vi "CIClose.vi"(11 "Camera data":variant) -> ()   [LabVIEW 2011]
uses:
  mkCameraData.ctl
  CameraConfig.ctl
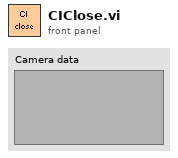
[diagram p1: front panel]
types:
  T1 = typedef "mkCameraData.ctl" = cluster{"Session":refnum<k11>, "Settings":T2}
  T2 = typedef "CameraConfig.ctl" = cluster{"Gain [1-4]":sgl, "Offset":i16, "Mode":i16, "ROIs":cluster{"X":i32, "Y":i32}[], "ROI Size":cluster{"X":i32, "Y":i32}, "Number of buffers":i32, "ZLUT Gain":sgl, "Display image size":cluster{"X":i32, "Y":i32}, "Use hardware multiple-ROI?":bool}
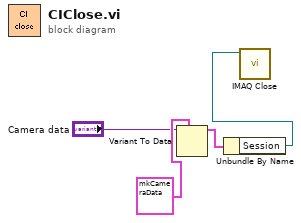
[diagram p0: block diagram]
diagram:
  n1 = Variant To Data(type=T1 {"Session"=refnum, "Settings"={"Gain [1-4]"=1.0, "Offset"=50, "Mode"=6, "ROIs"=[], "ROI Size"={"X"=0, "Y"=0}, "Number of buffers"=40, "ZLUT Gain"=1.0, "Display image size"={"X"=1280, "Y"=1024}, "Use hardware multiple-ROI?"=TRUE}} ("Camera data 2"), Variant="Camera data") -> (data=w2:T1)  [unwired: 1 in, 1 out]
  n2 = Unbundle By Name(w2) -> ("Session"=w1:refnum<k11>)
  n3 = call <vilib>:"IMAQ Close.vi"("IMAQ Session In"=w1) -> ()  [unwired: 10 in, 1 out]
